vi "update.assets.request.vi"(8 "error in":errorcluster, 10 "assets":refnum<class "asset.lvclass">[](array[class]), 11 "event":refnum<class "event.lvclass">) -> (0 "error out":errorcluster, 3 "request":string)   [LabVIEW 2020, in "event.lvclass"]
uses:
  event.lvclass
  asset/asset.lvclass
  event.lvclass/event.ctl
  asset/asset.lvclass/asset.ctl
  asset/rid.get.vi
  bfb2349f-e977-412d-987f-5a52b4c45808.vi
  <vilib>/JDP Science/JSONtext/Variant to JSON Text.vi
  <vilib>/JDP Science/JSONtext/LVClass Serializer/JSONtext LVClass Serializer.lvclass
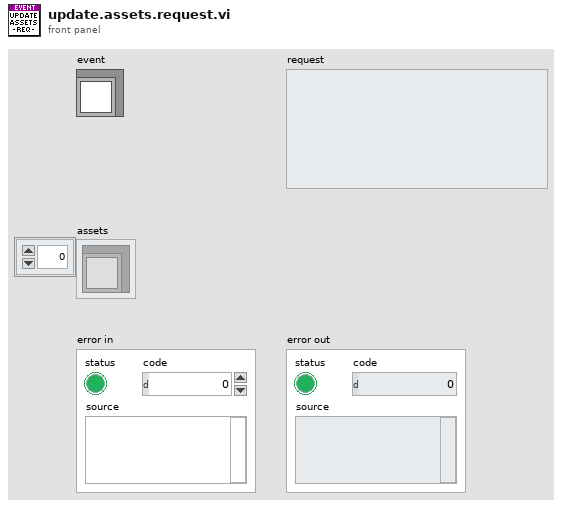
[diagram p1: front panel]
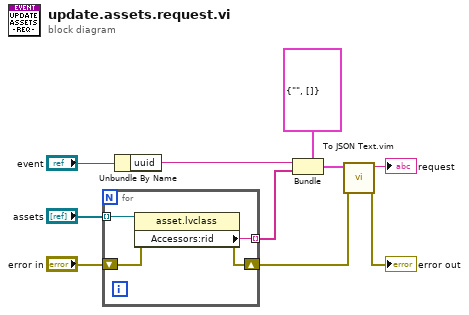
[diagram p0: block diagram]
diagram:
  n1 = for {
    tunnel: "assets" -> [w14] mode=indexing
    tunnel: [w13] -> w7 mode=indexing
    shift-right: [w11] -> w1
    shift-left: "error in" -> [w12]
    n2 = property class="asset.lvclass"(reference=w14, error in=w12) -> (error out=w11:errorcluster, "Accessors:rid"=w13:string)  [unwired: 1 out]
  }
  n3 = Unbundle By Name("event") -> ("uuid"=w8:string)
  n4 = Bundle(cluster=cluster{"uuid":string, "assetRids":string[]} {"uuid"="", "assetRids"=[]}, "uuid"=w8, "assetRids"=w7) -> (w5:cluster{"uuid":string, "assetRids":string[]})
  n5 = call "To JSON Text.vim"("error in (no error)"=w1, "Anything"=w5) -> ("error out"=→"error out":errorcluster, "<JSON>"=→"request":string)  [unwired: 8 in]
